vi "OP20B_Data.vi"() -> (2 "OP20B_004_PREACTUATION":T1)   [LabVIEW 2020]
uses:
  Controls/OP20B_DataCluster.ctl
panel:
  out "error out":errorcluster
  out "[CIRCLIP_POS_MIN]":dbl
  out "[CIRCLIP_POS]":dbl
  out "[CIRCLIP_POS_MAX]":dbl
  out "[CIRCLIP_POS_STATUS]":dbl
  out "[PREACTUATOR_TRAVEL_MIN]":dbl
  out "[PREACTUATOR_TRAVEL]":dbl
  out "[PREACTUATOR_TRAVEL_MAX]":dbl
  out "[PREACTUATOR_TRAVEL_STATUS]":dbl
  out "[CT]":dbl
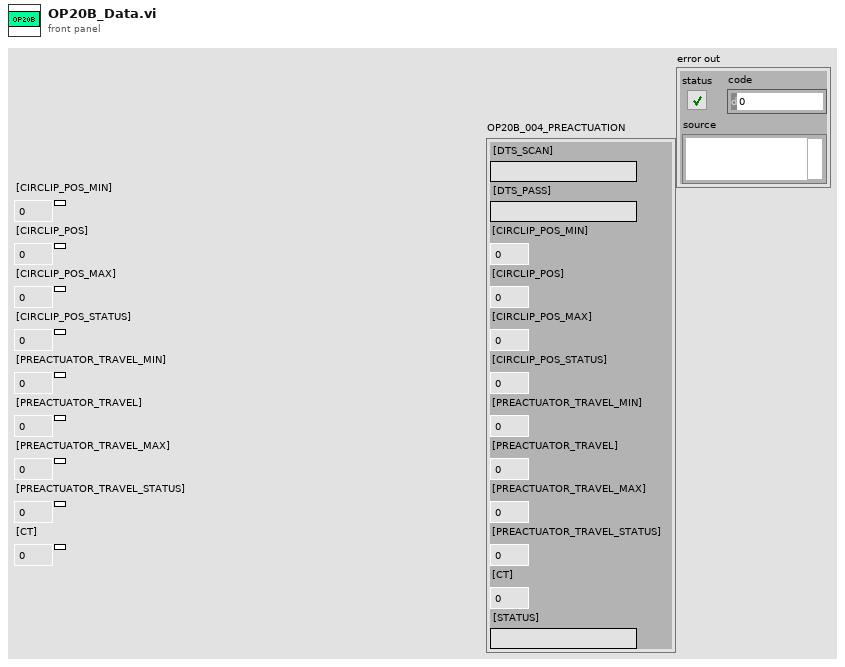
[diagram p1: front panel]
types:
  T1 = typedef "OP20B_DataCluster.ctl" = cluster{"[DTS_SCAN]":string, "[DTS_PASS]":string, "[CIRCLIP_POS_MIN]":dbl, "[CIRCLIP_POS]":dbl, "[CIRCLIP_POS_MAX]":dbl, "[CIRCLIP_POS_STATUS]":dbl, "[PREACTUATOR_TRAVEL_MIN]":dbl, "[PREACTUATOR_TRAVEL]":dbl, "[PREACTUATOR_TRAVEL_MAX]":dbl, "[PREACTUATOR_TRAVEL_STATUS]":dbl, "[CT]":dbl, "[STATUS]":string}
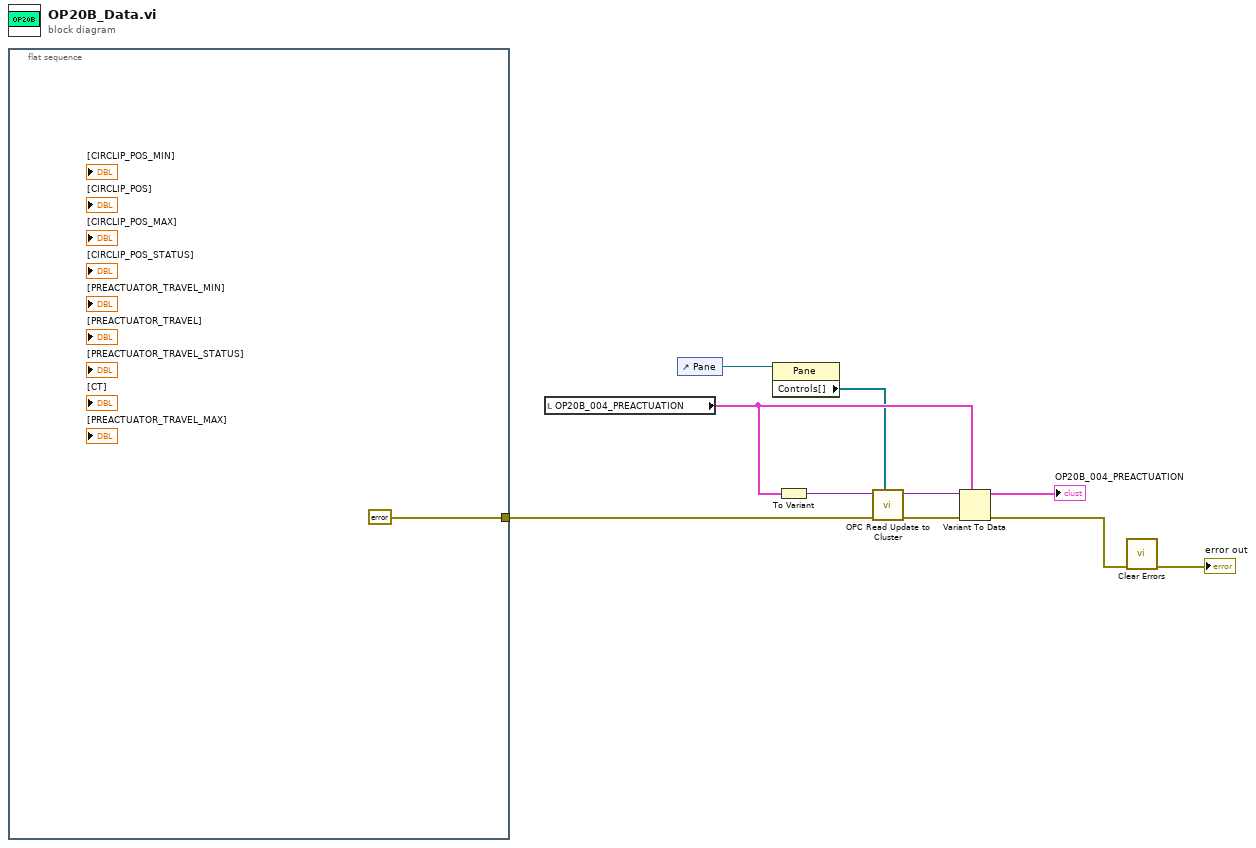
[diagram p0: block diagram]
diagram:
  n1 = flat-sequence {
    tunnel: [errorcluster {"status"=FALSE, "code"=0, "source"=""} ("error in (no error)")] -> w5
    frame #0 {
    }
  }
  n2 = local read "OP20B_004_PREACTUATION"() -> (w7:T1)
  n3 = control-ref of="Pane"() -> (w3:refnum<vi>)
  n4 = property class="Pane"(reference=w3) -> ("Controls[]"=w2:refnum<vi>[])  [unwired: 1 in, 2 out]
  n5 = To Variant(anything=w7) -> (Variant=w8:variant)
  n6 = call "OPC Read Update to Cluster.vi"("Controls[]"=w2, "error in (no error)"=w5, "Variant in"=w8) -> ("error out"=w9:errorcluster, "Variant out"=w10:variant)  [unwired: 7 in]
  n7 = Variant To Data(error in=w9, type=w7, Variant=w10) -> (data=→"OP20B_004_PREACTUATION":T1, error out=w4:errorcluster)
  n8 = call <vilib>:"Clear Errors.vi"("error in (no error)"=w4) -> ("error out"=→"error out":errorcluster)  [unwired: 5 in, 1 out]
